vi "Global 1.vi"() -> ()   [LabVIEW 2020]
panel:
  out "Msg":u32[](array[numeric])
  out "Buf":u8[](array[numeric]) format="%.0x"
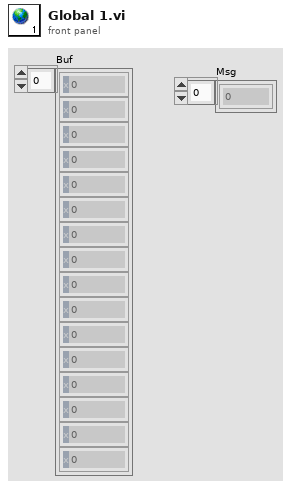
[diagram p1: front panel]
diagram:
